vi "Xbox Drive.vi"(7 "Right Side?":bool, 8 "Fire?":bool, 9 "Turn?":bool) -> (0 "Viewer Select":T1(ring)=enum."Ball Camera", 1 "Bridge Mode?":bool, 2 "Tank?":bool, 3 "Aligned?":bool, 5 "Shooter Is Front":bool)   [LabVIEW 2011]
uses:
  Team Code/Robot Global Data.vi
panel:
  in  "Bridge Mode Speed Reduction":dbl=2.0
  in  "Power Factor":dbl=3.0
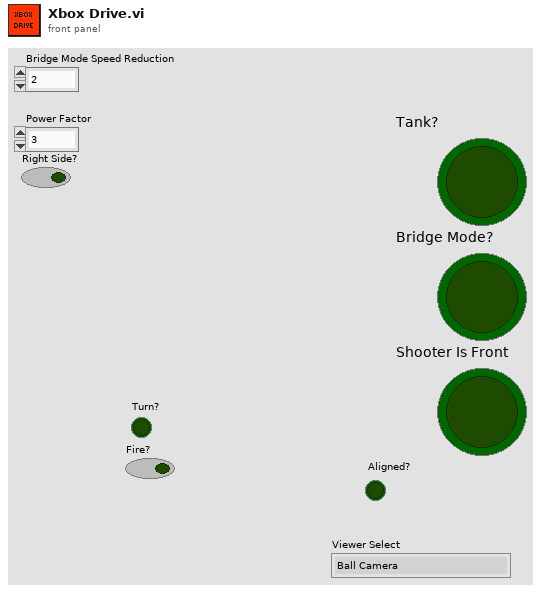
[diagram p1: front panel]
types:
  T1 = enum32{"Target Camera", "Target Camera Mask", "Ball Camera", "Kinect Skeleton"}
  T2 = typedef "WPI_JoystickButtonState.ctl" = cluster{"Button 1":bool, "Button 2":bool, "Button 3":bool, "Button 4":bool, "Button 5":bool, "Button 6":bool, "Button 7":bool, "Button 8":bool, "Button 9":bool, "Button 10":bool, "Button 11":bool, "Button 12":bool}
  T3 = cluster{"Buttons":T2, "Axes":cluster{"axis 1 (x)":dbl, "axis 2 (y)":dbl, "axis 3 (throttle)":dbl, "axis 4":dbl, "axis 5":dbl, "axis 6":dbl}}
  T4 = cluster{"Position":cluster{"X Angle":dbl, "Raw Y":dbl, "Raw X":dbl}, "Distance (ft)":dbl, "BB Angle":dbl}
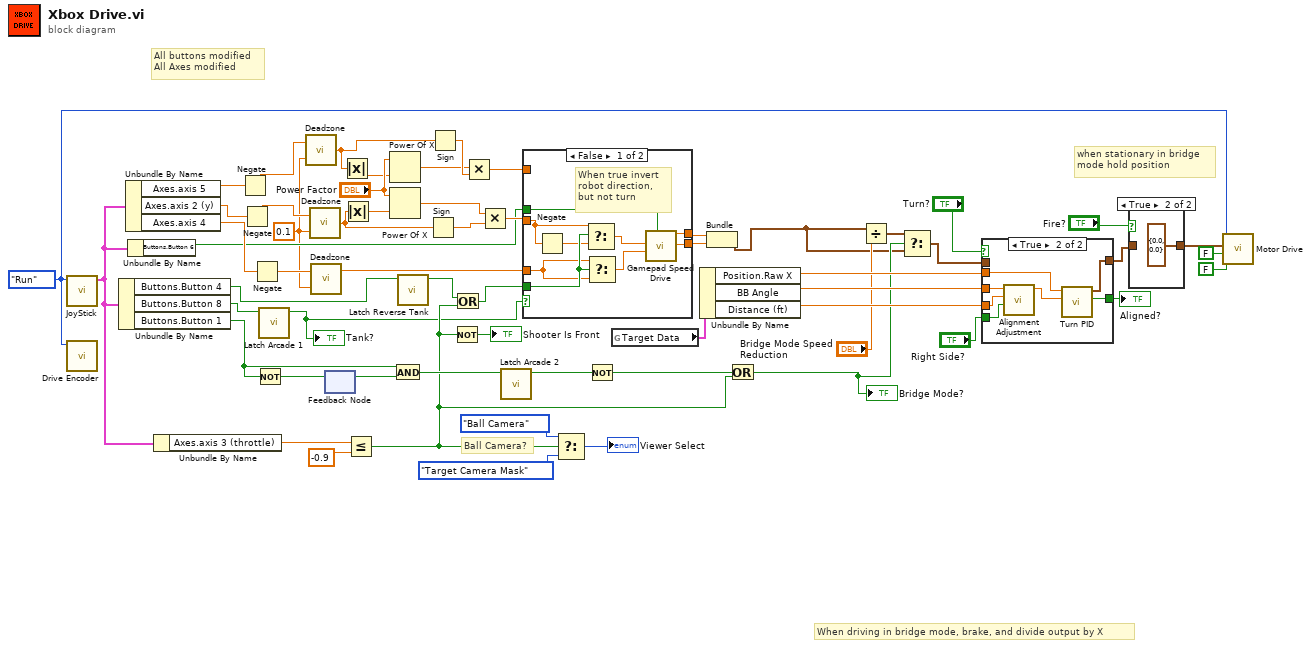
[diagram p0: block diagram]
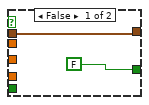
[diagram p3: hidden frame]
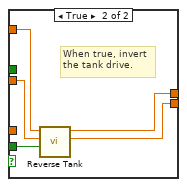
[diagram p4: hidden frame]
diagram:
  w28 = enum16{"Init", "Run", "End"}."Run" ("Enum")
  w14 = 0.1 ("Deadzone")
  # "All buttons modified\nAll Axes modified"
  # "Ball Camera?"
  # "when stationary in bridge \nmode hold position"
  # "When driving in bridge mode, brake, and divide output by X"
  n1 = call "JoyStick.vi"("Enum"=w28) -> ("JoyStick 1"=w18:T3)  [unwired: 7 in, 3 out]
  n2 = call "Drive Encoder.vi"("Enum"=w28) -> ()  [unwired: 10 in, 1 out]
  n3 = Unbundle By Name(w18) -> ("Buttons.Button 4"=w22:bool, "Buttons.Button 8"=w20:bool, "Buttons.Button 1"=w21:bool)
  n4 = Unbundle By Name(w18) -> ("Axes.axis 5"=w56:dbl, "Axes.axis 2 (y)"=w15:dbl, "Axes.axis 4"=w58:dbl)
  n5 = Unbundle By Name(w18) -> ("Buttons.Button 6"=w45:bool)
  n6 = Unbundle By Name(w18) -> ("Axes.axis 3 (throttle)"=w17:dbl)
  n7 = Negate(x=w56) -> (-x=w55:dbl)
  n8 = Negate(x=w15) -> (-x=w59:dbl)
  n9 = Negate(x=w58) -> (-x=w57:dbl)
  n10 = Not(x=w21) -> (.not. x?=w54:bool)
  n11 = call "Latch Arcade 1.vi"("Input"=w20) -> ("Latched"=w1:bool)  [unwired: 10 in]
  "Tank?" <- w1
  n12 = call "Deadzone.vi"("Deadzone"=w14, "Input"=w55) -> ("Output"=w27:dbl)
  n13 = call "Deadzone.vi"("Deadzone"=w14, "Input"=w59) -> ("Output"=w46:dbl)
  n14 = call "Deadzone.vi"("Deadzone"=w14, "Input"=w57) -> ("Output"=w44:dbl)
  n15 = feedback-in #1(w54) -> ()
  n16 = feedback #1() -> (w53:bool)  [unwired: 1 in]
  n17 = Absolute Value(x=w27) -> (abs(x)=w26:dbl)
  n18 = Absolute Value(x=w46) -> (abs(x)=w25:dbl)
  n19 = Less Or Equal?(x=w17, y=-0.9) -> (x <= y?=w3:bool)
  n20 = Power Of X(1:w26, 2:"Power Factor") -> (0:w24:dbl)
  n21 = Power Of X(1:w25, 2:"Power Factor") -> (0:w23:dbl)
  n22 = And(x=w21, y=w53) -> (x .and. y?=w33:bool)
  n23 = call "Latch Reverse Tank.vi"("Input"=w22) -> ("Latched"=w4:bool)  [unwired: 10 in]
  n24 = Sign(1:w46) -> (0:w47:dbl)
  n25 = Sign(1:w27) -> (0:w48:dbl)
  n26 = Not(x=w3) -> (.not. x?=→"Shooter Is Front":bool)
  n27 = Or(x=w4, y=w3) -> (x .or. y?=w2:bool)
  n28 = Multiply(x=w24, y=w48) -> (x*y=w50:dbl)
  n29 = Multiply(x=w23, y=w47) -> (x*y=w49:dbl)
  n30 = call "Latch Arcade 2.vi"("Input"=w33) -> ("Latched"=w16:bool)  [unwired: 10 in]
  n31 = case shown="False" w1 {
    tunnel: w45 -> [w65 _]
    tunnel: w49 -> [w61 w73]
    tunnel: w44 -> [w63 _]
    tunnel: [w68 w72] -> w43
    tunnel: [w67 w69] -> w42
    tunnel: w2 -> [w64 w71]
    tunnel: w50 -> [_ w70]
    frame False {
      # "When true invert robot direction, but not turn"
      n32 = Negate(x=w61) -> (-x=w62:dbl)
      n33 = Select(t=w61, s=w64, f=w62) -> (s? t:f=w60:dbl)
      n34 = Select(t=w63, s=w64, f=w63) -> (s? t:f=w66:dbl)
      n35 = call "Gamepad Speed Drive.vi"("Quick Turn"=w65, "Turn"=w66, "Speed"=w60) -> ("Right Output"=w67:dbl, "Left Output"=w68:dbl)  [unwired: 7 out]
    }
    frame True {
      # "When true, invert\nthe tank drive."
      n36 = call "Reverse Tank.vi"("Toggle Button"=w71, "Right Motor"=w73, "Left Motor"=w70) -> ("Right Motor"=w69:dbl, "Left Motor"=w72:dbl)  [unwired: 7 in]
    }
  }
  n37 = Select(t=T1."Ball Camera" ("Viewer Select"), s=w3, f=T1."Target Camera Mask" ("Viewer Select")) -> (s? t:f=→"Viewer Select":T1)
  n38 = Not(x=w16) -> (.not. x?=w13:bool)
  n39 = global read "Robot Global Data.vi" "Target Data"() -> (w31:T4)
  n40 = Unbundle By Name(w31) -> ("Position.Raw X"=w40:dbl, "BB Angle"=w39:dbl, "Distance (ft)"=w38:dbl)
  n41 = Bundle("Left Motor"=w43, "Right Motor"=w42) -> (w7:cluster{"Left Motor":dbl, "Right Motor":dbl})  [unwired: 1 out]
  n42 = Or(x=w13, y=w3) -> (x .or. y?=w8:bool)
  "Bridge Mode?" <- w8
  n43 = Divide(x=w7, y="Bridge Mode Speed Reduction") -> (x/y=w11:cluster{"Left Motor":dbl, "Right Motor":dbl})
  n44 = Select(t=w11, s=w8, f=w7) -> (s? t:f=w9:cluster{"Left Motor":dbl, "Right Motor":dbl})
  n45 = case shown="True" "Turn?" {
    tunnel: [w75 w79] -> w32
    tunnel: w9 -> [w75 _]
    tunnel: w40 -> [_ w76]
    tunnel: [FALSE w78] -> w41
    tunnel: "Right Side?" -> [_ w82]
    tunnel: w38 -> [_ w81]
    tunnel: w39 -> [_ w80]
    frame False {
    }
    frame True {
      n46 = call "Alignment Adjustment.vi"("Right Side of Field?"=w82, "Distance"=w81, "BB Angle"=w80) -> ("X Setpoint"=w77:dbl)  [unwired: 8 in]
      n47 = call "Turn PID.vi"("Setpoint X"=w77, "Current X"=w76) -> ("Aligned?"=w78:bool, "Motor Out"=w79:cluster{"output":dbl, dbl})  [unwired: 8 in]
    }
  }
  "Aligned?" <- w41
  n48 = case shown="True" "Fire?" {
    tunnel: w32 -> [w83 _]
    tunnel: [w83 cluster{"output":dbl, dbl} {"output"=0.0, 0.0} ("Motor Out")] -> w12
    frame False {
    }
    frame True {
    }
  }
  n49 = call "Motor Drive.vi"("Coast?"=FALSE, "Change Mode?"=FALSE, "Motor Input"=w12, "Enum"=w28) -> ()  [unwired: 8 in]
